vi "Distance To Angle.vi"(11 "Distance ft":dbl) -> (3 "Desired Angle":dbl)   [LabVIEW 2015]
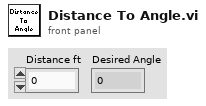
[diagram p1: front panel]
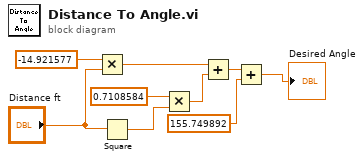
[diagram p0: block diagram]
diagram:
  n1 = Multiply(x=-14.921577, y="Distance ft") -> (x*y=w7:dbl)
  n2 = Square(x="Distance ft") -> (x^2=w6:dbl)
  n3 = Multiply(x=0.7108584, y=w6) -> (x*y=w8:dbl)
  n4 = Add(x=w7, y=w8) -> (x+y=w4:dbl)
  n5 = Add(x=w4, y=155.749892) -> (x+y=→"Desired Angle":dbl)
